vi "Untitled 1.vi"   [LabVIEW 2010]
uses:
  <vilib>/Waveform/DWDTOps.llb/DWDT Boolean Array to Digital.vi
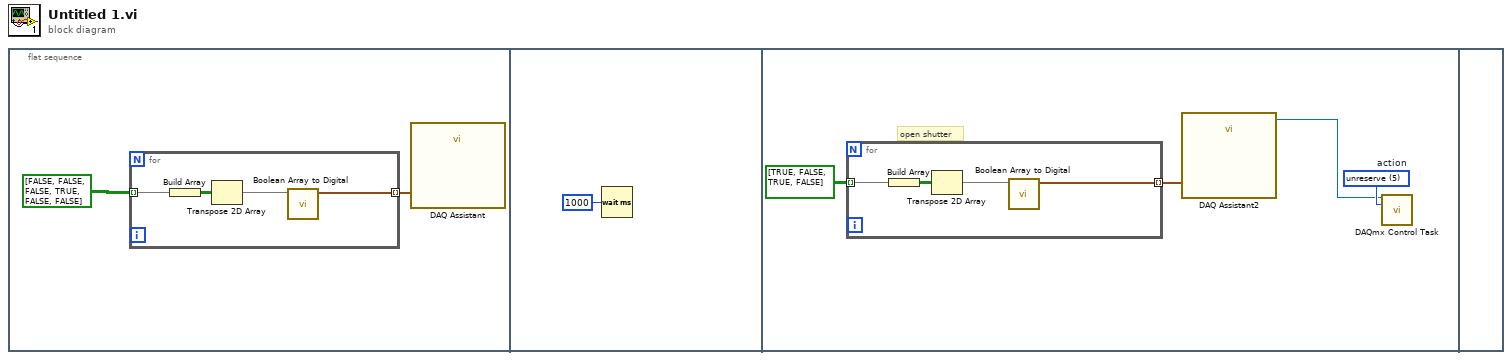
[diagram p0: block diagram]
diagram:
  n1 = flat-sequence {
    frame #0 {
      n2 = for {
        tunnel: bool[][] [[FALSE, FALSE, FALSE], [TRUE, FALSE, FALSE]] -> [w4] mode=indexing
        tunnel: [w5] -> w1 mode=indexing
        n3 = Build Array(w4) -> (w3:bool[][])
        n4 = Transpose 2D Array(2D array=w3) -> (transposed array=w6:bool[][])
        n5 = call-poly <vilib>:"Boolean Array to Digital.vi"("boolean array"=w6) -> ("digital waveform"=w5:digitalwaveform)  [unwired: 9 in, 1 out]
      }
      n6 = call "DAQ Assistant"("data"=w1) -> ()  [unwired: 17 in, 2 out]
    }
    frame #1 {
      n7 = Wait (ms)(milliseconds to wait=u32 1000) -> ()  [unwired: 1 out]
    }
    frame #2 {
      w9 = 5 items=["verify"=2, "reserve"=4, "commit"=3, "unreserve"=5, "abort"=6]  # action
      # "open shutter"
      n8 = for {
        tunnel: bool[][] [[TRUE, FALSE], [TRUE, FALSE]] -> [w13] mode=indexing
        tunnel: [w14] -> w11 mode=indexing
        n9 = Build Array(w13) -> (w12:bool[][])
        n10 = Transpose 2D Array(2D array=w12) -> (transposed array=w15:bool[][])
        n11 = call-poly <vilib>:"Boolean Array to Digital.vi"("boolean array"=w15) -> ("digital waveform"=w14:digitalwaveform)  [unwired: 9 in, 1 out]
      }
      n12 = call "DAQ Assistant2"("data"=w11) -> ("task out"=w8:refnum<k21>)  [unwired: 17 in, 1 out]
      n13 = call <vilib>:"DAQmx Control Task.vi"("task/channels in"=w8, "action"=w9) -> ()  [unwired: 12 in, 2 out]
    }
    frame #3 {
    }
  }
